vi "error stable.vi"(1 "Stable Current 1":dbl, 2 "Stable Current 2":dbl) -> (0 "Current error":dbl)   [LabVIEW 2016]
doc: "This is the calculation for the stable current contribution to the internal error"
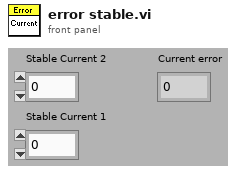
[diagram p1: front panel]
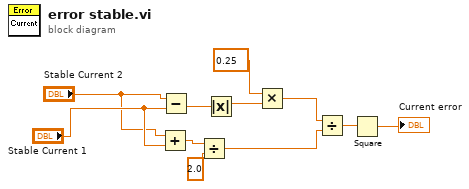
[diagram p0: block diagram]
diagram:
  n1 = Add(x="Stable Current 2", y="Stable Current 1") -> (x+y=w6:dbl)
  n2 = Subtract(x="Stable Current 2", y="Stable Current 1") -> (x-y=w1:dbl)
  n3 = Divide(x=w6, y=2.0) -> (x/y=w9:dbl)
  n4 = Absolute Value(x=w1) -> (abs(x)=w2:dbl)
  n5 = Multiply(x=0.25, y=w2) -> (x*y=w8:dbl)
  n6 = Divide(x=w8, y=w9) -> (x/y=w10:dbl)
  n7 = Square(x=w10) -> (x^2=→"Current error":dbl)
